vi "TMCM351-rotate.vi"(4 "执行？":bool, 5 "motor":u8(ring) items=["x", "y", "z"], 6 "错误输入":errorcluster caption="错误输入（无错误）", 7 "正转？":bool, 8 "Speed":i32=500 min=-2047 max=2048, 9 "com in":refnum<visa-resource-name>) -> (0 "错误输出":errorcluster, 3 "com out":refnum<visa-resource-name>)   [LabVIEW 2018]
uses:
  module_param.vi
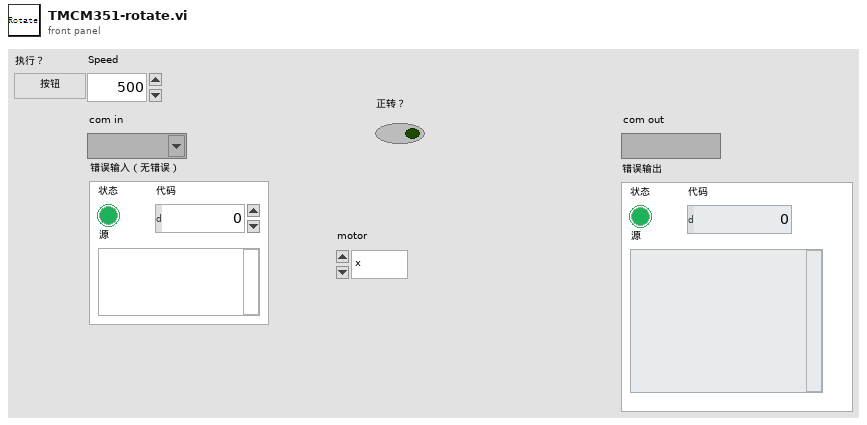
[diagram p1: front panel]
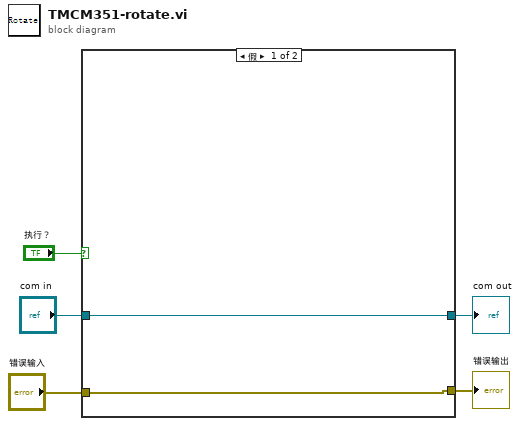
[diagram p0: block diagram]
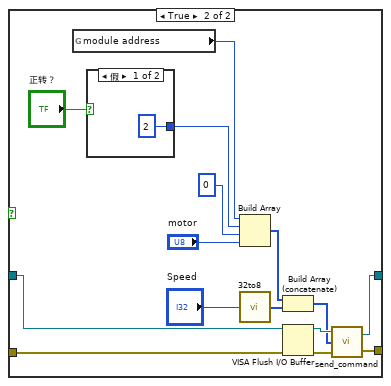
[diagram p2: hidden frame]
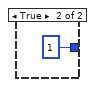
[diagram p3: hidden frame]
diagram:
  n1 = case shown="假" "执行？" {
    tunnel: "com in" -> [w7 w11]
    tunnel: "错误输入" -> [w6 w10]
    tunnel: [w7 w9] -> w2
    tunnel: [w6 w8] -> w1
    frame False {
    }
    frame True {
      n2 = global read "module_param.vi" "module address"() -> (w21:u8)
      n3 = case shown="假" "正转？" {
        tunnel: [u8 2 u8 1] -> w12
        frame False {
        }
        frame True {
        }
      }
      n4 = Build Array(w21, w12, u8 0, "motor") -> (w17:u8[])
      n5 = call "32to8.vi"("32data_in"="Speed") -> ("8Array"=w16:u8[])
      n6 = Build Array (concatenate)(w17, w16) -> (w15:u8[])
      n7 = VISA Flush I/O Buffer(VISA resource name=w11, error in (no error)=w10) -> (VISA resource name out=w19:refnum<visa-resource-name>, error out=w18:errorcluster)  [unwired: 1 in]
      n8 = call "send_command.vi"("错误输入"=w18, 3:w15, "com in"=w19) -> ("错误输出"=w8:errorcluster, "com out"=w9:refnum<visa-resource-name>)
    }
  }
  "com out" <- w2
  "错误输出" <- w1
